vi "14.2 Rotate Detect-2.vi"(8 "ErrI":errorcluster) -> ()   [LabVIEW 2016]
uses:
  <vilib>/vision/Image Controls.llb/IMAQ Image.ctl
  <vilib>/vision/NI_Vision_Development_Module.lvlib
panel:
  out "Tmplate":T1(plugin-control)
  out "Rotate Degree:":sgl format="%#_4g"
  out "IMG":T1(plugin-control)
  in  "Next":bool
  in  "Exit":bool
  # "Template Postion =0 Deg;\n\nRotate Degree compare to\ndegree 0 counter-clock wise."
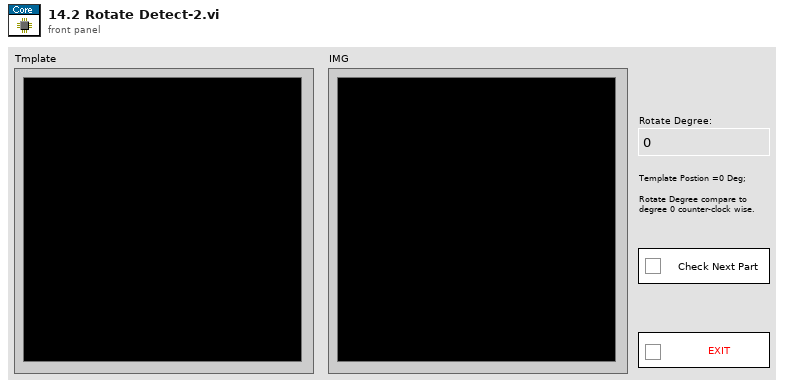
[diagram p1: front panel]
types:
  T1 = typedef "IMAQ Image.ctl" = refnum<image>
  T2 = cluster{"Tmp":T1, "Src":T1, "Radius":dbl, "Parts":string[], "Center":cluster{"X":sgl, "Y":sgl}, "Center0":cluster{"X":sgl, "Y":sgl}}
  T3 = typedef "IMAQ Circle" = cluster{"Center X":i32, "Center Y":i32, "Inner Radius":i32, "Outer Radius":i32, "Start Angle":dbl, "End Angle":dbl}
  T4 = typedef "Image Type" = u32
  T5 = typedef "ROI Descriptor" = cluster{"Global Rectangle":i32[], "Contours":cluster{"ID":enum32{"External", "Internal"}, "Type":u32, "Coordinates":i32[]}[]}
  T6 = cluster{"Center (Pixels)":cluster{"X":sgl, "Y":sgl}, "Radius (Pixels)":dbl, "Center (Real-World)":cluster{"X":sgl, "Y":sgl}, "Radius (Real-World)":dbl, "Roundness (Real-World)":dbl, "Average Strength":dbl, "Average SNR (dB)":dbl}
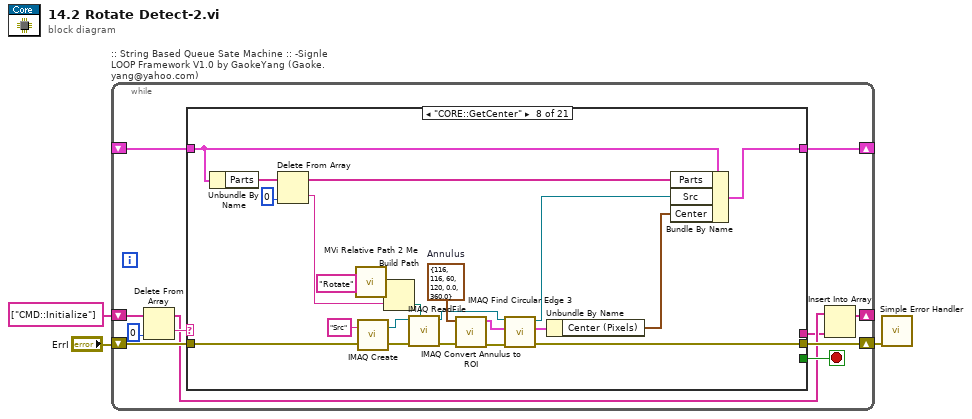
[diagram p0: block diagram]
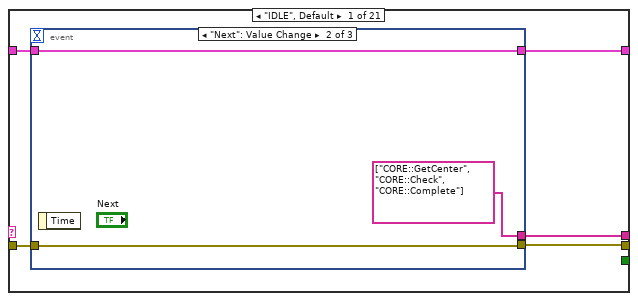
[diagram p2: hidden frame]
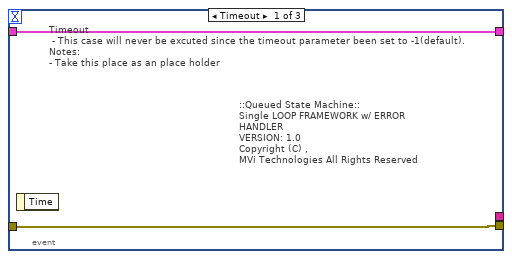
[diagram p3: hidden frame]
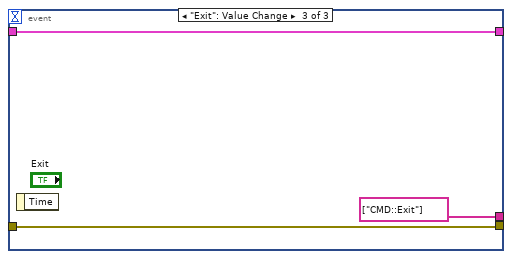
[diagram p4: hidden frame]
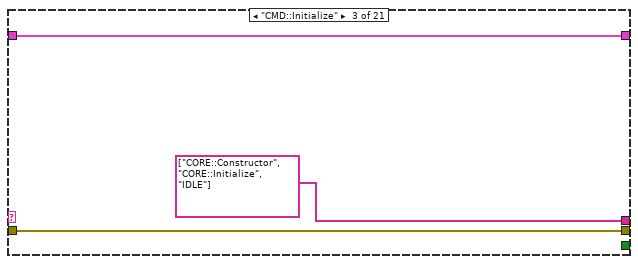
[diagram p6: hidden frame]
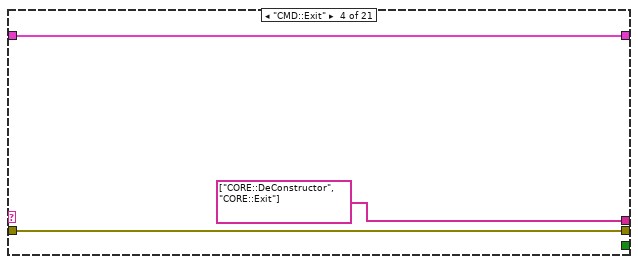
[diagram p7: hidden frame]
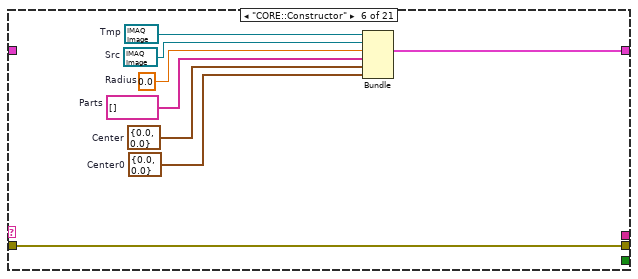
[diagram p9: hidden frame]
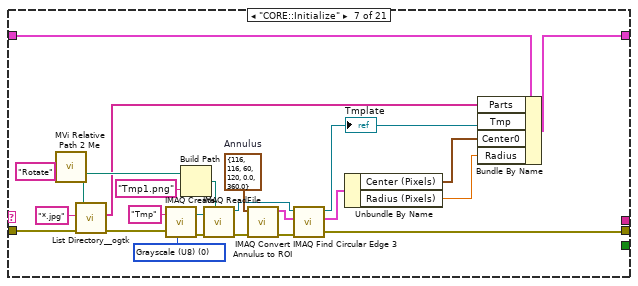
[diagram p10: hidden frame]
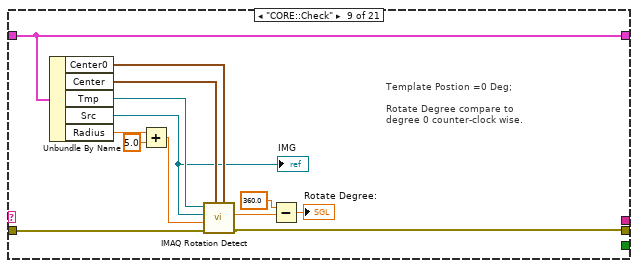
[diagram p11: hidden frame]
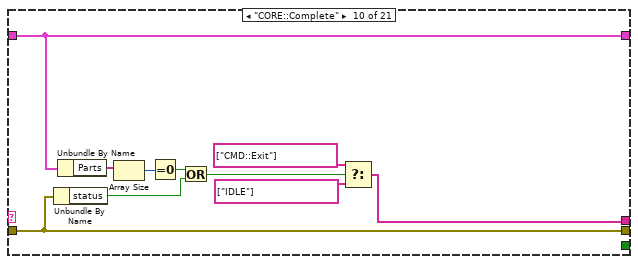
[diagram p12: hidden frame]
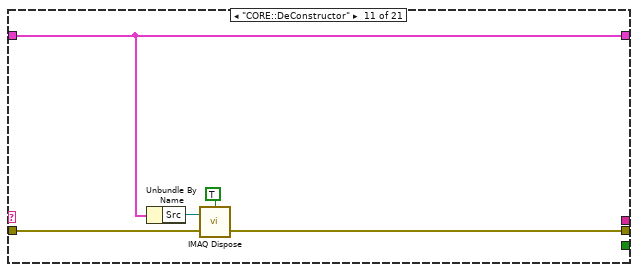
[diagram p13: hidden frame]
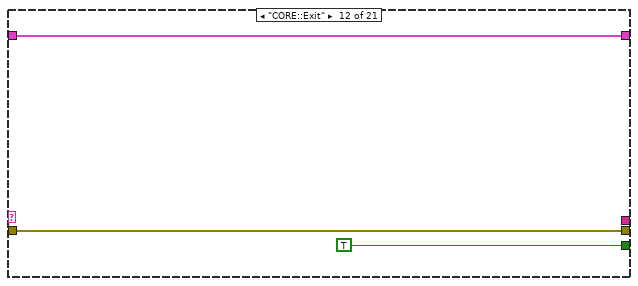
[diagram p14: hidden frame]
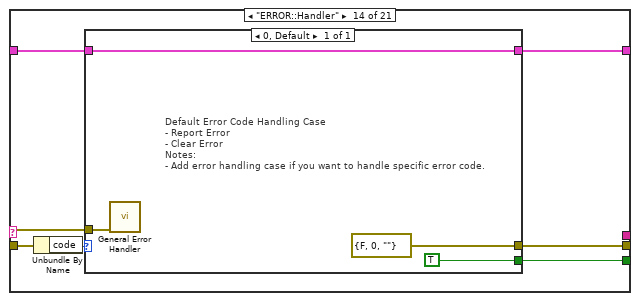
[diagram p16: hidden frame]
diagram:
  n1 = while ":: String Based Queue Sate Machine :: -Signle LOOP Framework V1.0 by GaokeYang (Gaoke.yang@yahoo.com)" {
    shift-right: [w11] -> w1
    shift-left: "ErrI" -> [w9]
    shift-right: [w13] -> _
    shift-left: _ -> [w12]
    shift-right: [w4] -> _
    shift-left: string[] ["CMD::Initialize"] -> [w10]
    stop <- w14 stop-if-true
    n2 = Delete From Array(array=w10, index=0) -> (deleted portion=w8:string, array with subset deleted=w6:string[])  [unwired: 1 in]
    n3 = case shown="\"CORE::GetCenter\"" w8 {
      tunnel: [w18 w29 w31 w34 w37 w44 w47 w82 w99 w110 w118 w120 w124 w127 w135 w137 w139 w142 w144 w146 w147] -> w11
      tunnel: [_ _ _ _ _ _ _ _ _ _ _ TRUE _ w126 _ _ _ _ _ _ _] -> w14
      tunnel: w9 -> [w19 w29 w31 w34 w37 w44 w56 w74 w103 w110 w119 w120 w124 w125 w135 w137 w139 w142 w144 w146 w147]
      tunnel: [w16 w28 w32 w35 w36 w45 w67 w84 w104 w111 w117 w121 w123 w128 w136 w138 w140 w141 w143 w145 w148] -> w13
      tunnel: w12 -> [w17 w28 w32 w35 w36 _ w68 w85 w104 w111 w117 w121 w123 w129 w136 w138 w140 w141 w143 w145 w148]
      tunnel: [w15 _ string[] ["CORE::Constructor", "CORE::Initialize", "IDLE"] string[] ["CORE::DeConstructor", "CORE::Exit"] _ _ _ _ _ w112 _ _ _ _ _ _ _ _ _ _ _] -> w5
      frame "IDLE", Default {
        n4 = event shown="[1] \"Next\": Value Change" {
          selector: _ -> [_ _ _]
          dyn-events: _ -> [_ _ _]
          timeout: _ -> [_ _ _]
          tunnel: [w21 w24 w27] -> w18
          tunnel: w19 -> [w21 w24 w27]
          tunnel: [w20 w23 w26] -> w16
          tunnel: w17 -> [w20 w23 w26]
          tunnel: [_ string[] ["CORE::GetCenter", "CORE::Check", "CORE::Complete"] string[] ["CMD::Exit"]] -> w15
          event Timeout {
            # "Timeout\n - This case will never be excuted since the timeout parameter been set to -1(default).\nNotes:\n- Take this place as an place holder"
            # "::Queued State Machine::\nSingle LOOP FRAMEWORK w/ ERROR HANDLER\nVERSION: 1.0\nCopyright (C) ,\nMVi Technologies All Rights Reserved"
            n5 = event-data() -> ()  [unwired: 1 in, 1 out]
          }
          event "Next": Value Change {
            n6 = event-data() -> ()  [unwired: 1 in, 1 out]
          }
          event "Exit": Value Change {
            n7 = event-data() -> ()  [unwired: 1 in, 1 out]
          }
        }
      }
      frame "-------- Commands ---------" {
      }
      frame "CMD::Initialize" {
      }
      frame "CMD::Exit" {
      }
      frame "------------ Core ------------" {
      }
      frame "CORE::Constructor" {
        w38 = 0.0  # Radius
        w39 = cluster{"X":sgl, "Y":sgl} {"X"=0.0, "Y"=0.0}  # Center0
        w40 = cluster{"X":sgl, "Y":sgl} {"X"=0.0, "Y"=0.0}  # Center
        w42 = T1 refnum  # Src
        w41 = string[] []  # Parts
        w43 = T1 refnum  # Tmp
        n8 = Bundle("Tmp"=w43, "Src"=w42, "Radius"=w38, "Parts"=w41, "Center"=w40, "Center0"=w39) -> (w45:T2)  [unwired: 1 in]
      }
      frame "CORE::Initialize" {
        w61 = T3 {"Center X"=116, "Center Y"=116, "Inner Radius"=60, "Outer Radius"=120, "Start Angle"=0.0, "End Angle"=360.0}  # Annulus
        w62 = T4 0 items=["Grayscale (U8)", "Grayscale (I16)", "Grayscale (SGL)", "Complex (CSG)", "RGB (U32)", "HSL (U32)", "RGB (U64)", "Grayscale (U16)"] ("Image Type")
        n9 = call "MVi Relative Path 2 Me.vi"("Relative Path"="Rotate" ("name or relative path")) -> ("Appended Dir"=w54:path)  [unwired: 5 in, 1 out]
        n10 = call "List Directory__ogtk.vi"("error in (no error)"=w56, "pattern"="*.jpg", "directory path"=w54) -> ("error out"=w55:errorcluster, "file names"=w51:string[])  [unwired: 1 in, 2 out]
        n11 = call "IMAQ Create"("Image Name"="Tmp", "Image Type"=w62, "error in (no error)"=w55) -> ("Src"=w66:T1, "error out"=w65:errorcluster)  [unwired: 2 in]
        n12 = Build Path(base path=w54, name or relative path="Tmp1.png") -> (appended path=w52:path)
        n13 = call "IMAQ ReadFile"("File Path"=w52, "error in (no error)"=w65, "Image"=w66) -> ("error out"=w59:errorcluster, "Image Out"=w58:T1)  [unwired: 4 in, 3 out]
        n14 = call "IMAQ Convert Annulus to ROI"("error in (no error)"=w59, "Annulus"=w61) -> ("error out"=w57:errorcluster, "ROI Descriptor"=w60:T5)  [unwired: 7 in]
        n15 = call "IMAQ Find Circular Edge 3"("error in (no error)"=w57, "ROI Descriptor"=w60, "Image"=w58) -> ("error out"=w47:errorcluster, "Fitted Circle"=w49:T6, "Image Out"=w50:T1)  [unwired: 4 in, 2 out]
        "Tmplate" <- w50
        n16 = Unbundle By Name(w49) -> ("Center (Pixels)"=w48:cluster{"X":sgl, "Y":sgl}, "Radius (Pixels)"=w46:dbl)
        n17 = Bundle By Name(cluster=w68, "Parts"=w51, "Tmp"=w50, "Center0"=w48, "Radius"=w46) -> (w67:T2)
      }
      frame "CORE::GetCenter" {
        w80 = T3 {"Center X"=116, "Center Y"=116, "Inner Radius"=60, "Outer Radius"=120, "Start Angle"=0.0, "End Angle"=360.0}  # Annulus
        n18 = Unbundle By Name(w85) -> ("Parts"=w83:string[])
        n19 = Delete From Array(array=w83, index=0) -> (deleted portion=w88:string, array with subset deleted=w86:string[])  [unwired: 1 in]
        n20 = call "MVi Relative Path 2 Me.vi"("Relative Path"="Rotate" ("name or relative path")) -> ("Appended Dir"=w90:path)  [unwired: 5 in, 1 out]
        n21 = call "IMAQ Create"("Image Name"="Src", "error in (no error)"=w74) -> ("Src"=w72:T1, "error out"=w73:errorcluster)  [unwired: 3 in]
        n22 = Build Path(base path=w90, name or relative path=w88) -> (appended path=w87:path)
        n23 = call "IMAQ ReadFile"("File Path"=w87, "error in (no error)"=w73, "Image"=w72) -> ("error out"=w77:errorcluster, "Image Out"=w76:T1)  [unwired: 4 in, 3 out]
        n24 = call "IMAQ Convert Annulus to ROI"("error in (no error)"=w77, "Annulus"=w80) -> ("error out"=w81:errorcluster, "ROI Descriptor"=w79:T5)  [unwired: 7 in]
        n25 = call "IMAQ Find Circular Edge 3"("error in (no error)"=w81, "ROI Descriptor"=w79, "Image"=w76) -> ("error out"=w82:errorcluster, "Fitted Circle"=w78:T6, "Image Out"=w71:T1)  [unwired: 4 in, 2 out]
        n26 = Unbundle By Name(w78) -> ("Center (Pixels)"=w70:cluster{"X":sgl, "Y":sgl})
        n27 = Bundle By Name(cluster=w85, "Parts"=w86, "Src"=w71, "Center"=w70) -> (w84:T2)
      }
      frame "CORE::Check" {
        # "Template Postion =0 Deg;\n\nRotate Degree compare to\ndegree 0 counter-clock wise."
        n28 = Unbundle By Name(w104) -> ("Center0"=w100:cluster{"X":sgl, "Y":sgl}, "Center"=w101:cluster{"X":sgl, "Y":sgl}, "Tmp"=w102:T1, "Src"=w98:T1, "Radius"=w94:dbl)
        "IMG" <- w98
        n29 = Add(x=w94, y=5.0) -> (x+y=w92:dbl)
        n30 = call "IMAQ Rotation Detect"("Reference Center"=w100, "Image 2 Center"=w101, "error in (no error)"=w103, "Radius"=w92, "Image 2"=w98, "Reference Image"=w102) -> ("error out"=w99:errorcluster, "Angle (deg)"=w96:dbl)  [unwired: 3 in, 1 out]
        n31 = Subtract(x=360.0, y=w96) -> (x-y=→"Rotate Degree:":dbl)
      }
      frame "CORE::Complete" {
        n32 = Unbundle By Name(w110) -> ("status"=w106:bool)
        n33 = Unbundle By Name(w111) -> ("Parts"=w109:string[])
        n34 = Array Size(array=w109) -> (size(s)=w108:i32)
        n35 = Equal To 0?(x=w108) -> (x = 0?=w107:bool)
        n36 = Or(x=w107, y=w106) -> (x .or. y?=w105:bool)
        n37 = Select(t=string[] ["CMD::Exit"], s=w105, f=string[] ["IDLE"]) -> (s? t:f=w112:string[])
      }
      frame "CORE::DeConstructor" {
        n38 = Unbundle By Name(w117) -> ("Src"=w116:T1)
        n39 = call "IMAQ Dispose"("All Images? (No)"=TRUE, "Image"=w116, "error in (no error)"=w119) -> ("error out"=w118:errorcluster)  [unwired: 3 in]
      }
      frame "CORE::Exit" {
      }
      frame "-------- Error Handle--------" {
      }
      frame "ERROR::Handler" {
        n40 = Unbundle By Name(w125) -> ("code"=w130:i32)
        n41 = case shown="0, Default" w130 {
          tunnel: [w134] -> w128
          tunnel: w129 -> [w134]
          tunnel: [errorcluster {"status"=FALSE, "code"=0, "source"=""} ("error out")] -> w127
          tunnel: [TRUE] -> w126
          tunnel: w125 -> [w132]
          frame 0, Default {
            # "Default Error Code Handling Case\n- Report Error\n- Clear Error \nNotes:\n- Add error handling case if you want to handle specific error code."
            n42 = call <vilib>:"General Error Handler.vi"("error in (no error)"=w132) -> ()  [unwired: 10 in, 5 out]
          }
        }
      }
      frame "------------  GUI  ------------" {
      }
      frame "GUI::Initialize" {
      }
      frame "GUI::SetCusor" {
      }
      frame "GUI::SetMenu" {
      }
      frame "------------ USER -----------" {
      }
      frame "USER::Case1" {
      }
      frame "USER::Case2" {
      }
    }
    n43 = Insert Into Array(array=w6, new element=w5) -> (w4:string[])  [unwired: 1 in]
  }
  n44 = call <vilib>:"Simple Error Handler.vi"("error in (no error)"=w1) -> ()  [unwired: 4 in, 5 out]
